vi "Start Module.vi"(8 "error in (no error)":errorcluster, 11 "Run as Singleton? (F)":bool) -> (0 "error out":errorcluster, 1 "Wait for Event Sync?":bool, 2 "LGP5 Acquisition Broadcast Events":T1, 3 "Module ID":i32)   [LabVIEW 2018, in "LGP5 Acquisition.lvlib"]
doc: "Launches the Module Main.vi.\n_____\nBased on Delacor QMH Project Template 4.1.0.59."
uses:
  LGP5 Acquisition.lvlib
  Broadcast Events--cluster.ctl
  Did Init Argument--cluster.ctl
  Status Updated Argument--cluster.ctl
  Error Reported Argument--cluster.ctl
  Stop Argument--cluster.ctl
  Get Module Execution Status Argument--cluster.ctl
  Module Running State--enum.ctl
  <vilib>/Delacor/Delacor QMH/Libraries/Cloneable Module Admin_class/Delacor_lib_QMH_Cloneable Module Admin.lvclass
  C:/Program Files (x86)/National Instruments/LabVIEW 2018/vi.lib/Delacor/Delacor QMH/Libraries/Module Admin_class/Delacor_lib_QMH_Module Admin.lvclass
  <vilib>/Delacor/Delacor QMH/Libraries/Cloneable Module Admin_class/Delacor_lib_QMH_Cloneable Module Admin.lvclass/Delacor_lib_QMH_Cloneable Module Admin.ctl
  <vilib>/Delacor/Delacor QMH/Libraries/Module Admin_class/Delacor_lib_QMH_Module Admin.lvclass/Delacor_lib_QMH_Module Admin.ctl
  <vilib>/Delacor/Delacor QMH/Libraries/Cloneable Module Admin_class/Delacor_lib_QMH_Set Module ID.vi
  <vilib>/Delacor/Delacor QMH/Libraries/Module Admin_class/Delacor_lib_QMH_Set External Launch.vi
  <vilib>/Utility/error.llb/Error Cluster From Error Code.vi
  <vilib>/ErrorRing/Error Ring.xnode
  Clone Registration/Clone Registration.lvlib
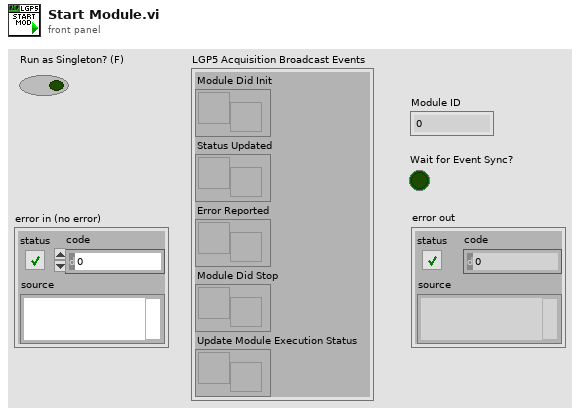
[diagram p1: front panel]
types:
  T1 = typedef "LGP5 Acquisition.lvlib/Broadcast Events--cluster.ctl" = cluster{"Module Did Init":refnum<user-event>, "Status Updated":refnum<user-event>, "Error Reported":refnum<user-event>, "Module Did Stop":refnum<user-event>, "Update Module Execution Status":refnum<user-event>}
  T2 = typedef "LGP5 Acquisition.lvlib/Module Running State--enum.ctl" = enum16{"Not Running", "Running as Cloneable", "Running as Singleton"}
  T3 = enum32{"Bad", "Idle", "Run top level", "Running"}
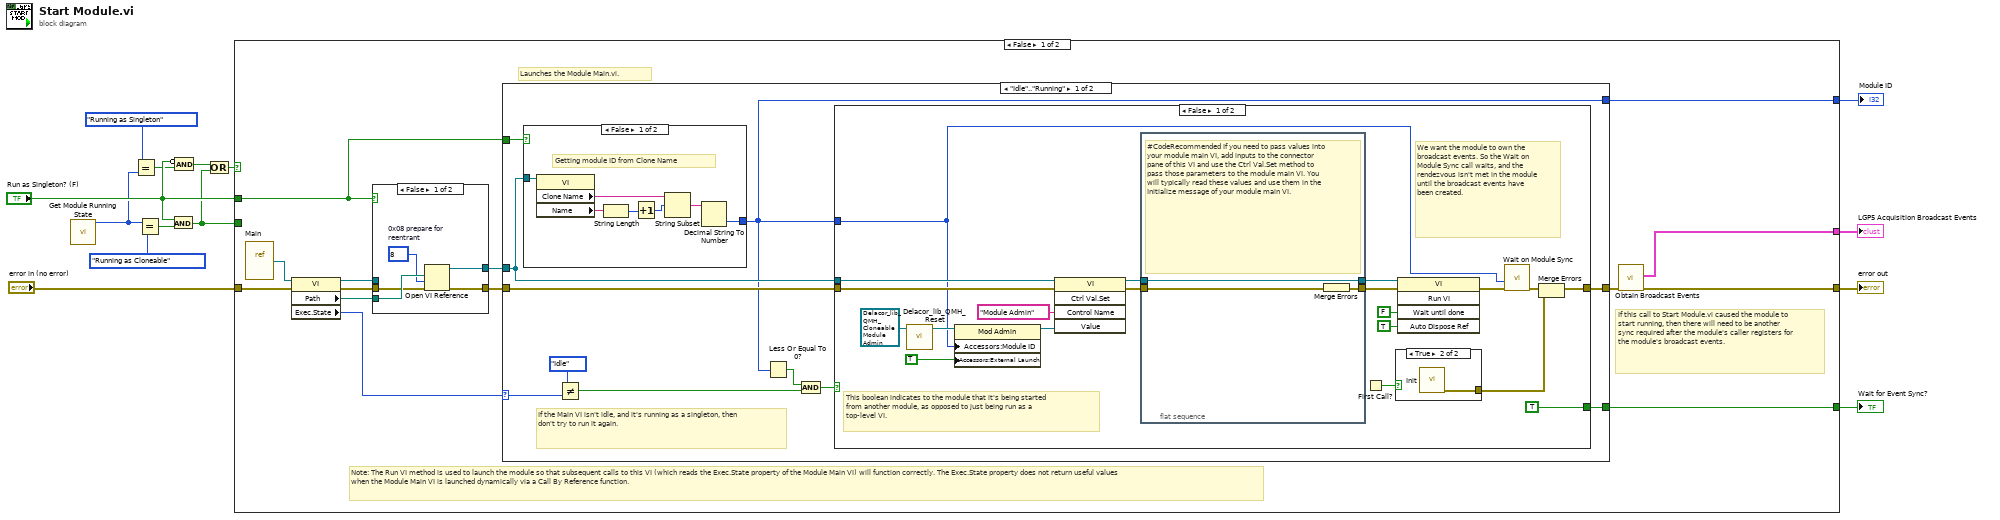
[diagram p0: block diagram]
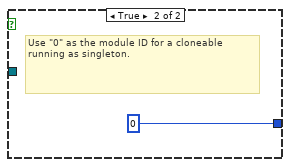
[diagram p3: hidden frame]
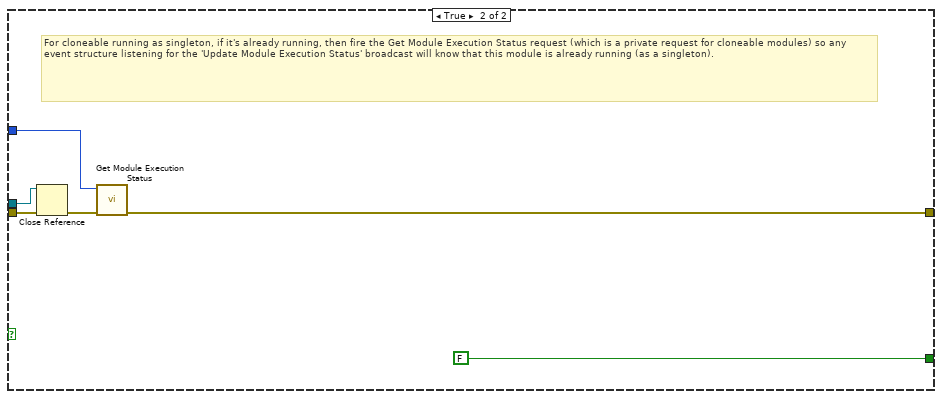
[diagram p5: hidden frame]
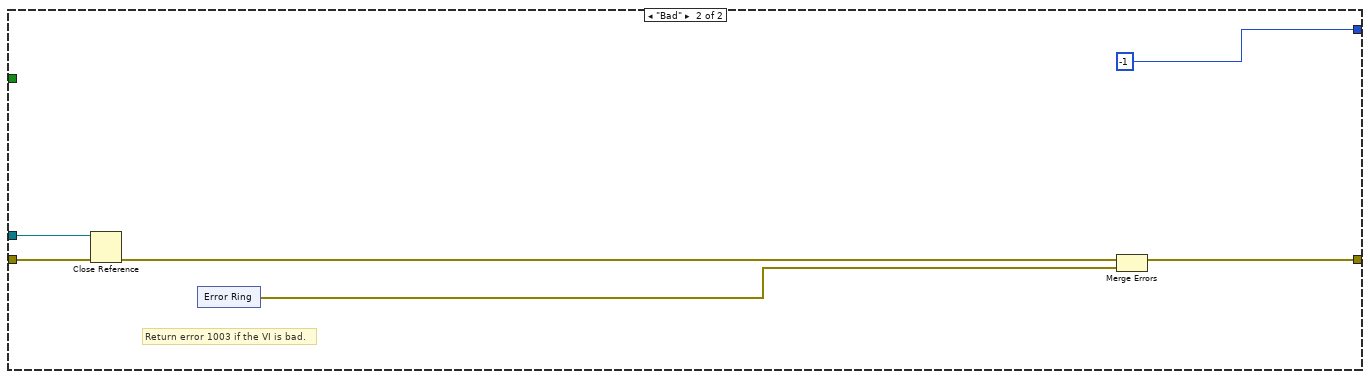
[diagram p6: hidden frame]
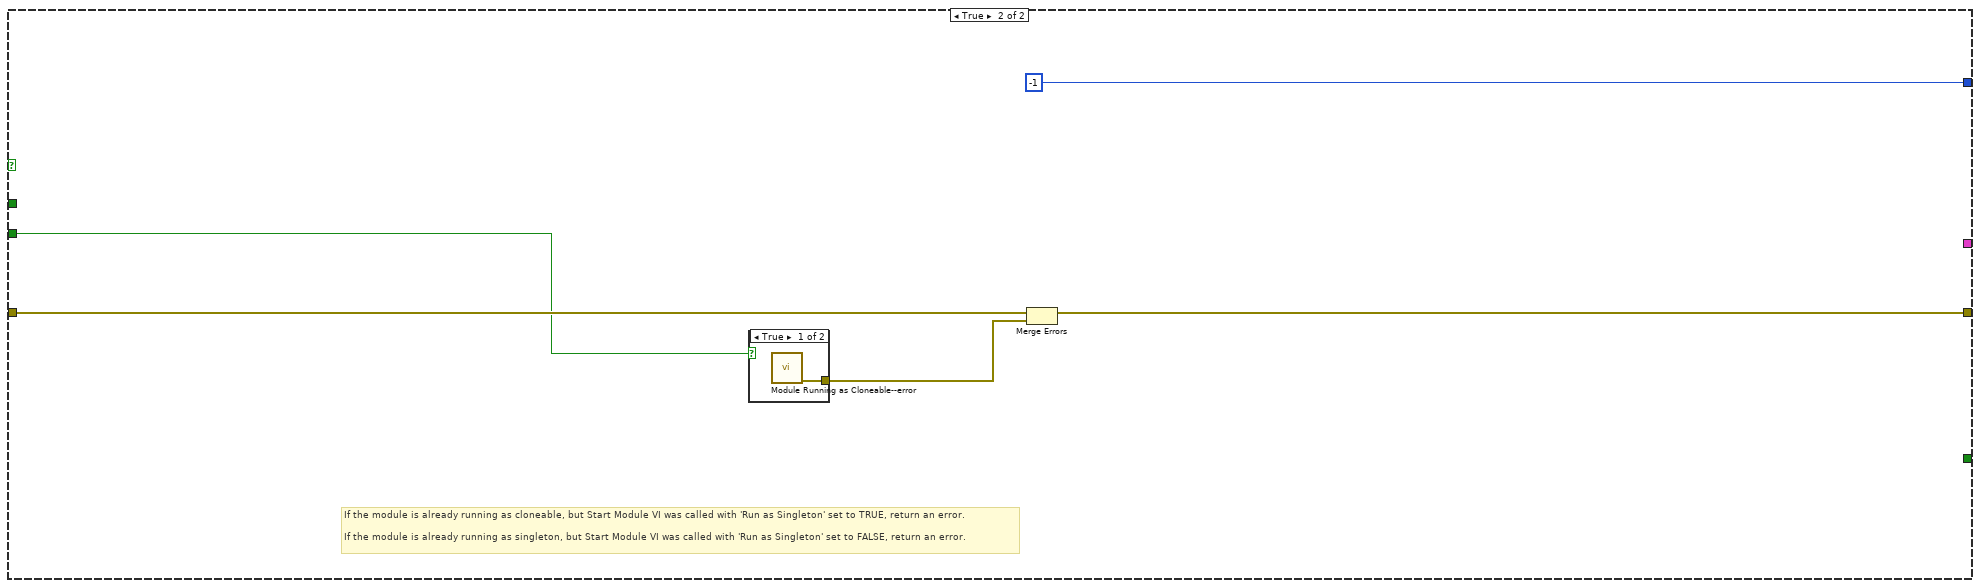
[diagram p7: hidden frame]
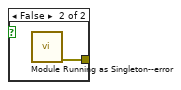
[diagram p8: hidden frame]
diagram:
  n1 = call "Get Module Running State.vi"() -> ("Module Running State"=w3:T2)  [unwired: 11 in]
  n2 = Equal?(x=Module_Running_State--enum."Running as Singleton", y=w3) -> (x = y?=w4:bool)
  n3 = Equal?(x=w3, y=Module_Running_State--enum."Running as Cloneable") -> (x = y?=w8:bool)
  n4 = And(x="Run as Singleton? (F)", y=w8) -> (x .and. y?=w1:bool)
  n5 = Compound Arithmetic op=AND(invert "Run as Singleton? (F)", w4) -> (w6:bool)
  n6 = Or(x=w6, y=w1) -> (x .or. y?=w7:bool)
  n7 = case shown="False" w7 {
    tunnel: "error in (no error)" -> [w28 w99]
    tunnel: [w26 w98] -> w13
    tunnel: [w25 _] -> w12
    tunnel: [w24 _] -> w11
    tunnel: [w20 -1] -> w10
    tunnel: "Run as Singleton? (F)" -> [w16 _]
    tunnel: w1 -> [_ w95]
    frame False {
      # "Note: The Run VI method is used to launch the module so that subsequent calls to this VI (which reads the Exec.State property of the Module Main VI) will function correctly. The Exec.State property does not return useful values when the Module Main VI is launched dynamically via a Call By Reference function."
      # "If this call to Start Module.vi caused the module to start running, then there will need to be another sync required after the module's caller registers for the module's broadcast events."
      # "Launches the Module Main.vi."
      n8 = vi-ref "Main.vi"() -> (w19:refnum<vi>)
      n9 = property class="VI"(reference=w19, error in=w28) -> (reference out=w15:refnum<vi>, error out=w22:errorcluster, "Path"=w23:path, "Exec.State"=w17:T3)
      n10 = case shown="False" w16 {
        tunnel: w23 -> [w33 _]
        tunnel: w22 -> [w32 w35]
        tunnel: [w31 w35] -> w21
        tunnel: [w29 w34] -> w18
        tunnel: w15 -> [_ w34]
        frame False {
          w30 = 8  # 0x08 prepare for reentrant
          n11 = Open VI Reference(vi path=w33, options=w30, error in (no error)=w32) -> (vi reference=w29:refnum<vi>, error out=w31:errorcluster)  [unwired: 3 in]
        }
        frame True {
        }
      }
      n12 = case shown="\"Idle\"..\"Running\"" w17 {
        selector: w17 -> [w42 _]
        tunnel: w21 -> [w46 w90]
        tunnel: w18 -> [w44 w89]
        tunnel: [w43 w87] -> w27
        tunnel: [w45 _] -> w24
        tunnel: [w37 -1] -> w20
        tunnel: w16 -> [w36 _]
        frame "Idle".."Running" {
          # "If the Main VI isn't idle, and it's running as a singleton, then don't try to run it again."
          n13 = case shown="False" w36 {
            tunnel: w44 -> [w53 _]
            tunnel: [w47 0] -> w37
            frame False {
              # "Getting module ID from Clone Name"
              n14 = property class="VI"(reference=w53) -> ("Clone Name"=w50:string, "Name"=w49:string)  [unwired: 1 in, 2 out]
              n15 = String Length(string=w49) -> (length=w51:i32)
              n16 = Increment(x=w51) -> (x+1=w52:i32)
              n17 = String Subset ("Getting module ID from Clone Name")(string=w50, offset (0)=w52) -> (substring=w48:string)  [unwired: 1 in]
              n18 = Decimal String To Number(string=w48) -> (number=w47:i32)  [unwired: 2 in, 1 out]
            }
            frame True {
              # "Use \"0\" as the module ID for a cloneable running as singleton."
            }
          }
          n19 = Not Equal?(x=T3."Idle", y=w42) -> (x != y?=w40:bool)
          n20 = Less Or Equal To 0?(x=w37) -> (x <= 0?=w38:bool)
          n21 = And(x=w38, y=w40) -> (x .and. y?=w39:bool)
          n22 = case shown="False" w39 {
            tunnel: w46 -> [w74 w83]
            tunnel: [TRUE FALSE] -> w45
            tunnel: w44 -> [w67 w80]
            tunnel: [w65 w79] -> w43
            tunnel: w37 -> [w59 w82]
            frame False {
              # "We want the module to own the broadcast events. So the Wait on Module Sync call waits, and the rendezvous isn't met in the module until the broadcast events have been created."
              # "This boolean indicates to the module that it's being started from another module, as opposed to just being run as a top-level VI."
              n23 = call-dynamic "Delacor_lib_QMH_Reset.vi"("Mod Admin in"=refnum<class "Delacor_lib_QMH_Cloneable Module Admin.lvclass"> refnum) -> ("Mod Admin out"=w63:refnum<class "Delacor_lib_QMH_Cloneable Module Admin.lvclass">)  [unwired: 9 in, 1 out]
              n24 = property class="Mod Admin"(reference=w63, "Accessors:Module ID"=w59, "Accessors:External Launch"=TRUE) -> (reference out=w62:refnum<class "Delacor_lib_QMH_Cloneable Module Admin.lvclass">)  [unwired: 1 in, 1 out]
              n25 = invoke class="VI" method="Ctrl Val.Set"(reference=w67, error in=w74, "Control Name"="Module Admin", "Value"=w62) -> (reference out=w58:refnum<vi>, error out=w57:errorcluster)  [unwired: 1 in, 3 out]
              n26 = flat-sequence {
                tunnel: w58 -> [w77]
                tunnel: [w77] -> w56
                tunnel: w57 -> [w76]
                tunnel: [w75] -> w55
                frame #0 {
                  # "#CodeRecommended If you need to pass values into your module main VI, add inputs to the connector pane of this VI and use the Ctrl Val.Set method to pass those parameters to the module main VI. You will typically read these values and use them in the Initialize message of your module main VI."
                  n27 = Merge Errors(w76) -> (w75:errorcluster)
                }
              }
              n28 = First Call?() -> (First Call?: T/F=w66:bool)
              n29 = case shown="True" w66 {
                tunnel: [_ w78] -> w64
                frame False {
                }
                frame True {
                  n30 = call "Init.vi"() -> ("error out"=w78:errorcluster)  [unwired: 8 in, 3 out]
                }
              }
              n31 = invoke class="VI" method="Run VI"(reference=w56, error in=w55, "Wait until done"=FALSE ("Wait Until Done"), "Auto Dispose Ref"=TRUE ("Auto Dispose Reference")) -> (error out=w71:errorcluster)  [unwired: 1 in, 4 out]
              n32 = call "Wait on Module Sync.vi"("error in (no error)"=w71, "Module ID"=w59) -> ("error out"=w70:errorcluster)  [unwired: 9 in]
              n33 = Merge Errors(w70, w64) -> (w65:errorcluster)
            }
            frame True {
              # "For cloneable running as singleton, if it's already running, then fire the Get Module Execution Status request (which is a private request for cloneable modules) so any event structure listening for the 'Update Module Execution Status' broadcast will know that this module is already running (as a singleton)."
              n34 = Close Reference(reference=w80, error in (no error)=w83) -> (error out=w81:errorcluster)
              n35 = call "Get Module Execution Status.vi"("error in (no error)"=w81, "Module ID"=w82) -> ("error out"=w79:errorcluster)  [unwired: 9 in]
            }
          }
        }
        frame "Bad" {
          # "Return error 1003 if the VI is bad."
          n36 = Close Reference(reference=w89, error in (no error)=w90) -> (error out=w88:errorcluster)
          n37 = xnode "Error Ring"() -> ("error out"=w86:errorcluster)
          n38 = Merge Errors(w88, w86) -> (w87:errorcluster)
        }
      }
      n39 = call "Obtain Broadcast Events.vi"("error in (no error)"=w27) -> ("error out"=w26:errorcluster, "LGP5 Acquisition Broadcast Events"=w25:T1)  [unwired: 9 in]
    }
    frame True {
      # "If the module is already running as cloneable, but Start Module VI was called with 'Run as Singleton' set to TRUE, return an error.\n\nIf the module is already running as singleton, but Start Module VI was called with 'Run as Singleton' set to FALSE, return an error."
      n40 = case shown="True" w95 {
        tunnel: [w100 w101] -> w96
        frame True {
          n41 = call "Module Running as Cloneable--error.vi"() -> ("error out"=w100:errorcluster)  [unwired: 11 in]
        }
        frame False {
          n42 = call "Module Running as Singleton--error.vi"() -> ("error out"=w101:errorcluster)  [unwired: 11 in]
        }
      }
      n43 = Merge Errors(w99, w96) -> (w98:errorcluster)
    }
  }
  "error out" <- w13
  "LGP5 Acquisition Broadcast Events" <- w12
  "Wait for Event Sync?" <- w11
  "Module ID" <- w10
